vi "tsapp_get_error_description.vi"(8 "error in":errorcluster, 10 "ACount":i32, 11 "路径输入":path) -> (0 "error out":errorcluster, 2 "ErrDes":string, 3 "路径输出":path)   [LabVIEW 2014]
doc: "Obtain fault description"
uses:
  <vilib>/Utility/importsl/GetValueByPointer/GetValueByPointer.xnode
  <vilib>/Utility/importsl/GetValueByPointer/datatype.ctl
panel:
  out "ACode":i32
  out "ErrDesAddr":i64
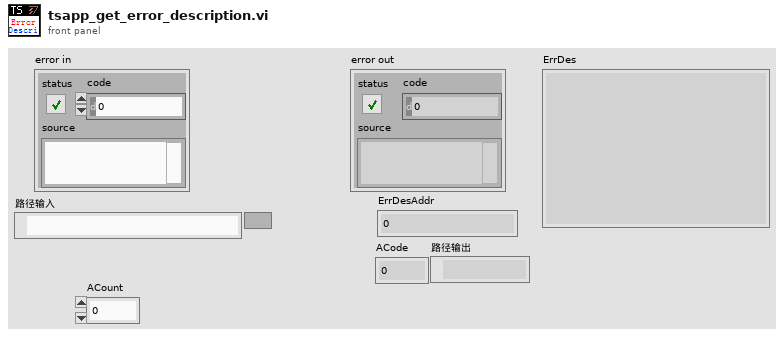
[diagram p1: front panel]
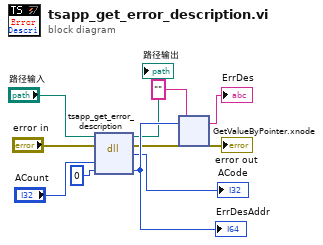
[diagram p0: block diagram]
diagram:
  n1 = dll-call lib="D:/Program Files (x86)/TOSUN/TSMaster/bin/libTSMaster.dll" fn="tsapp_get_error_description"(path in="路径输入", error in="error in", "ACode"="ACount", "ErrDesAddr"=u64 0) -> (path out=→"路径输出":path, error out=w5:errorcluster, "Code"=→"ACode":i32, "ErrDesAddr"=w8:u64)  [unwired: 2 in]
  "ErrDesAddr" <- w8
  n2 = xnode "GetValueByPointer.xnode"("Pointer"=w8, "InputType"="", "ErrorIn"=w5) -> ("Output"=→"ErrDes":string, "ErrorOut"=→"error out":errorcluster)  [unwired: 1 in]
